vi "SEEK_Recipe_Range_Validation.vi"(0 "SeekAmplitudeLoopC1":i32, 1 "SeekFreqLimitHigh":i32, 2 "SeekRampTime":i32, 3 "SeekPhaseloopI":i32, 5 "SeekFreqOffset":i32, 7 "MemoryClearBeforeSeek":i32, 9 "SeekTime":i32, 12 "SeekAmplitudeLoopC2":i32, 13 "SeekPhaseloopCF":i32, 14 "SeekFreqLimitLow":i32) -> (4 "String":string)   [LabVIEW 2017]
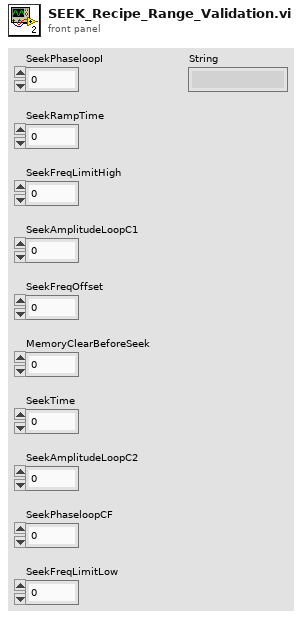
[diagram p1: front panel]
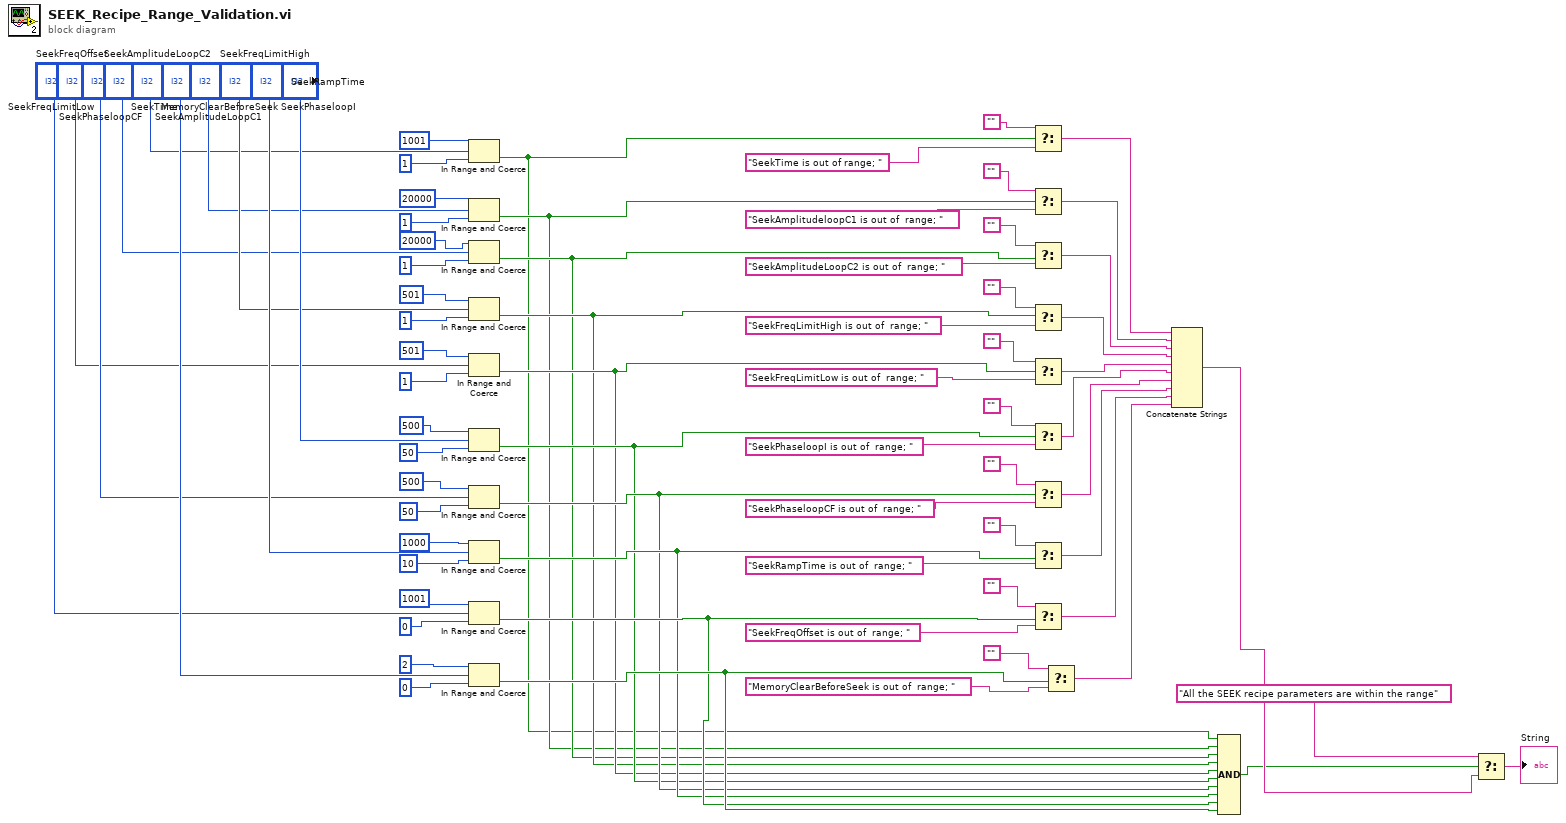
[diagram p0: block diagram]
diagram:
  n1 = In Range and Coerce(upper limit=1001, x="SeekTime", lower limit=1) -> (In Range?=w61:bool)  [unwired: 1 out]
  n2 = In Range and Coerce(upper limit=20000, x="SeekAmplitudeLoopC1", lower limit=1) -> (In Range?=w62:bool)  [unwired: 1 out]
  n3 = In Range and Coerce(upper limit=20000, x="SeekAmplitudeLoopC2", lower limit=1) -> (In Range?=w63:bool)  [unwired: 1 out]
  n4 = In Range and Coerce(upper limit=501, x="SeekFreqLimitHigh", lower limit=1) -> (In Range?=w64:bool)  [unwired: 1 out]
  n5 = In Range and Coerce(upper limit=501, x="SeekFreqLimitLow", lower limit=1) -> (In Range?=w65:bool)  [unwired: 1 out]
  n6 = In Range and Coerce(upper limit=500, x="SeekPhaseloopI", lower limit=50) -> (In Range?=w66:bool)  [unwired: 1 out]
  n7 = In Range and Coerce(upper limit=500, x="SeekPhaseloopCF", lower limit=50) -> (In Range?=w67:bool)  [unwired: 1 out]
  n8 = In Range and Coerce(upper limit=1000, x="SeekRampTime", lower limit=10) -> (In Range?=w68:bool)  [unwired: 1 out]
  n9 = In Range and Coerce(upper limit=1001, x="SeekFreqOffset", lower limit=0) -> (In Range?=w69:bool)  [unwired: 1 out]
  n10 = In Range and Coerce(upper limit=2, x="MemoryClearBeforeSeek", lower limit=0) -> (In Range?=w70:bool)  [unwired: 1 out]
  n11 = Select(t="", s=w61, f="SeekTime is out of range; ") -> (s? t:f=w51:string)
  n12 = Select(t="", s=w62, f="SeekAmplitudeloopC1 is out of  range; ") -> (s? t:f=w52:string)
  n13 = Select(t="", s=w63, f="SeekAmplitudeLoopC2 is out of  range; ") -> (s? t:f=w53:string)
  n14 = Select(t="", s=w64, f="SeekFreqLimitHigh is out of  range; ") -> (s? t:f=w54:string)
  n15 = Select(t="", s=w65, f="SeekFreqLimitLow is out of  range; ") -> (s? t:f=w55:string)
  n16 = Select(t="", s=w66, f="SeekPhaseloopI is out of  range; ") -> (s? t:f=w56:string)
  n17 = Select(t="", s=w67, f="SeekPhaseloopCF is out of  range; ") -> (s? t:f=w57:string)
  n18 = Select(t="", s=w68, f="SeekRampTime is out of  range; ") -> (s? t:f=w58:string)
  n19 = Select(t="", s=w69, f="SeekFreqOffset is out of  range; ") -> (s? t:f=w59:string)
  n20 = Select(t="", s=w70, f="MemoryClearBeforeSeek is out of  range; ") -> (s? t:f=w60:string)
  n21 = Concatenate Strings(w51, w52, w53, w54, w55, w56, w57, w58, w59, w60) -> (w73:string)
  n22 = Compound Arithmetic op=AND(w61, w62, w63, w64, w65, w66, w67, w68, w69, w70) -> (w71:bool)
  n23 = Select(t="All the SEEK recipe parameters are within the range", s=w71, f=w73) -> (s? t:f=→"String":string)
